vi "Test Base Config File as Directory Path.vi"(8 "error in (no error)":errorcluster, 11 "Base Test In":refnum<class "Base Dev Test.lvclass">) -> (0 "error out":errorcluster, 3 "Base Test Out":refnum<class "Base Dev Test.lvclass">)   [LabVIEW 2020, in "Base Dev Test.lvclass"]
uses:
  Base Dev Test.lvclass
  C:/Program Files (x86)/National Instruments/LabVIEW 2020/vi.lib/Astemes/LUnit/Test Case.lvclass
  source/Framework/Base/Base.lvclass
  <vilib>/Astemes/LUnit/Test Case.lvclass/Test Case.ctl
  <vilib>/Astemes/LUnit/LUnit Assertion Result.lvclass/LUnit Assertion Result.ctl
  <vilib>/Astemes/LUnit/LUnit Test Case Result.lvclass/LUnit Test Case Result.ctl
  <vilib>/Astemes/LUnit/LUnit Method Result.lvclass/LUnit Method Result.ctl
  <vilib>/Astemes/LUnit/Palette/Fail.vi
  <vilib>/Astemes/LUnit/Palette/Pass.vi
  <vilib>/Astemes/LUnit/Set Assertion Type.vi
  <vilib>/Astemes/LUnit/Add test result.vi
  <vilib>/Astemes/LUnit/LUnit Write Passed.vi
  <vilib>/Astemes/LUnit/LUnit Write Message.vi
  <vilib>/Astemes/LUnit/LUnit Write Description.vi
  <vilib>/Astemes/LUnit/LUnit Write Assertion Type.vi
  <vilib>/Astemes/LUnit/LUnit Record Assertion Result.vi
  <vilib>/Astemes/LUnit/LUnit Aggregate Assertion Results.vi
  <vilib>/Astemes/LUnit/Assertion Result/LUnit Read Status.vi
  <vilib>/Astemes/LUnit/LUnit Read Message.vi
  <vilib>/Astemes/LUnit/LUnit Read Description.vi
  <vilib>/Astemes/LUnit/Method Result/LUnit Merge Status.vi
  <vilib>/Astemes/LUnit/LUnit Concatenate result strings.vi
  <vilib>/Astemes/LUnit/LUnit Assertion Result.lvclass
  <vilib>/Astemes/LUnit/Test Case.lvclass
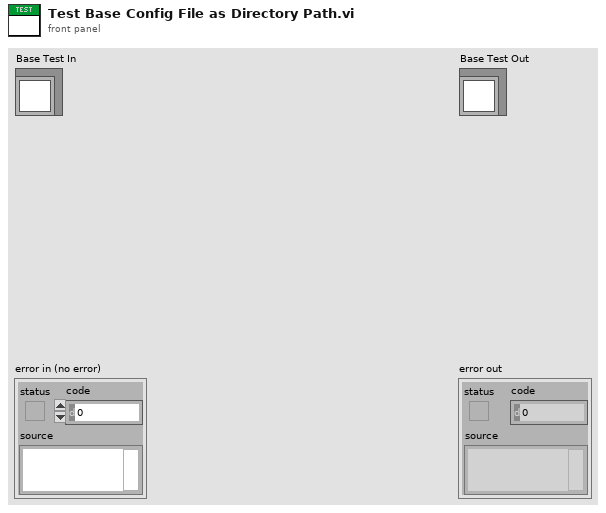
[diagram p1: front panel]
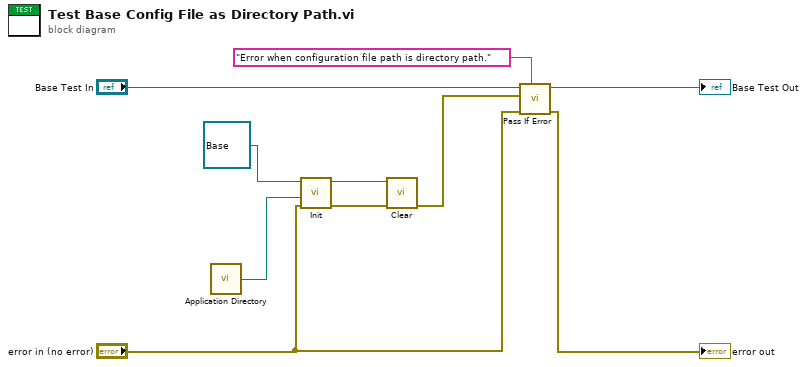
[diagram p0: block diagram]
diagram:
  n1 = call <vilib>:"Application Directory.vi"() -> ("Application Directory"=w7:path)
  n2 = call-dynamic "Init.vi"("error in (no error)"="error in (no error)", "Config File Path"=w7, "Base In"=refnum<class "Base.lvclass"> refnum ("Application.lvclass")) -> ("error out"=w8:errorcluster, "Base Out"=w9:refnum<class "Base.lvclass">)  [unwired: 7 in]
  n3 = call-dynamic "Clear.vi"("error in (no error)"=w8, "Base In"=w9) -> ("error out"=w5:errorcluster)  [unwired: 9 in]
  n4 = call <vilib>:"Pass If Error.vi"("Description"="Error when configuration file path is directory path.", "error in (no error)"="error in (no error)", "Assert error"=w5, "LUnit Test Case In"="Base Test In") -> ("error out"=→"error out":errorcluster, "LUnit Test Case Out"=→"Base Test Out":refnum<class "Base Dev Test.lvclass">)  [unwired: 6 in]
